vi "energy_list.vi"(10 "list_peak_energies":string[][](array[string]), 11 "List Calibration":T2[](array[typedef]) {"Select Line" items=["Ka1", "Ka2", "Kb1", "La1", "La2", "Lb1", "Lb2", "Lg1"]; "Select Element" items=["Li", "Be", "B", "C", "N", "O", "F", "Ne", "Na", "Mg", "Al", "Si", "P", "S", "Cl", "Ar", "K", "Ca", "Sc", "Ti", "V", "Cr", "Mn", "Fe", "Co", "Ni", "Cu", "Zn", "Ga", "Ge", "As", "Se", "Br", "Kr", "Rb", "Sr", "Y", "Zr", "Nb", "Mo", "Tc", "Ru", "Rh", "Pd", "Ag", "Cd", "In", "Sn", "Sb", "Te", "I", "Xe", "Cs", "Ba", "La", "Ce", "Pr", "Nd", "Pm", "Sm", "Eu", "Gd", "Tb", "Dy", "Ho", "Er", "Tm", "Yb", "Lu", "Hf", "Ta", "W", "Re", "Os", "Ir", "Pt", "Au", "Hg", "Tl", "Pb", "Bi", "Po", "At", "Rn", "Fr", "Ra", "Ac", "Th", "Pa", "U", "Np", "Pu", "Am"]}) -> (1 "Check":bool[](array[boolean]), 2 "to calibrate":T1, 3 "List Calibration Out":T2[](array[typedef]) {"Select Line" items=["Ka1", "Ka2", "Kb1", "La1", "La2", "Lb1", "Lb2", "Lg1"]; "Select Element" items=["Li", "Be", "B", "C", "N", "O", "F", "Ne", "Na", "Mg", "Al", "Si", "P", "S", "Cl", "Ar", "K", "Ca", "Sc", "Ti", "V", "Cr", "Mn", "Fe", "Co", "Ni", "Cu", "Zn", "Ga", "Ge", "As", "Se", "Br", "Kr", "Rb", "Sr", "Y", "Zr", "Nb", "Mo", "Tc", "Ru", "Rh", "Pd", "Ag", "Cd", "In", "Sn", "Sb", "Te", "I", "Xe", "Cs", "Ba", "La", "Ce", "Pr", "Nd", "Pm", "Sm", "Eu", "Gd", "Tb", "Dy", "Ho", "Er", "Tm", "Yb", "Lu", "Hf", "Ta", "W", "Re", "Os", "Ir", "Pt", "Au", "Hg", "Tl", "Pb", "Bi", "Po", "At", "Rn", "Fr", "Ra", "Ac", "Th", "Pa", "U", "Np", "Pu", "Am"]})   [LabVIEW 2023]
uses:
  control/calib.ctl
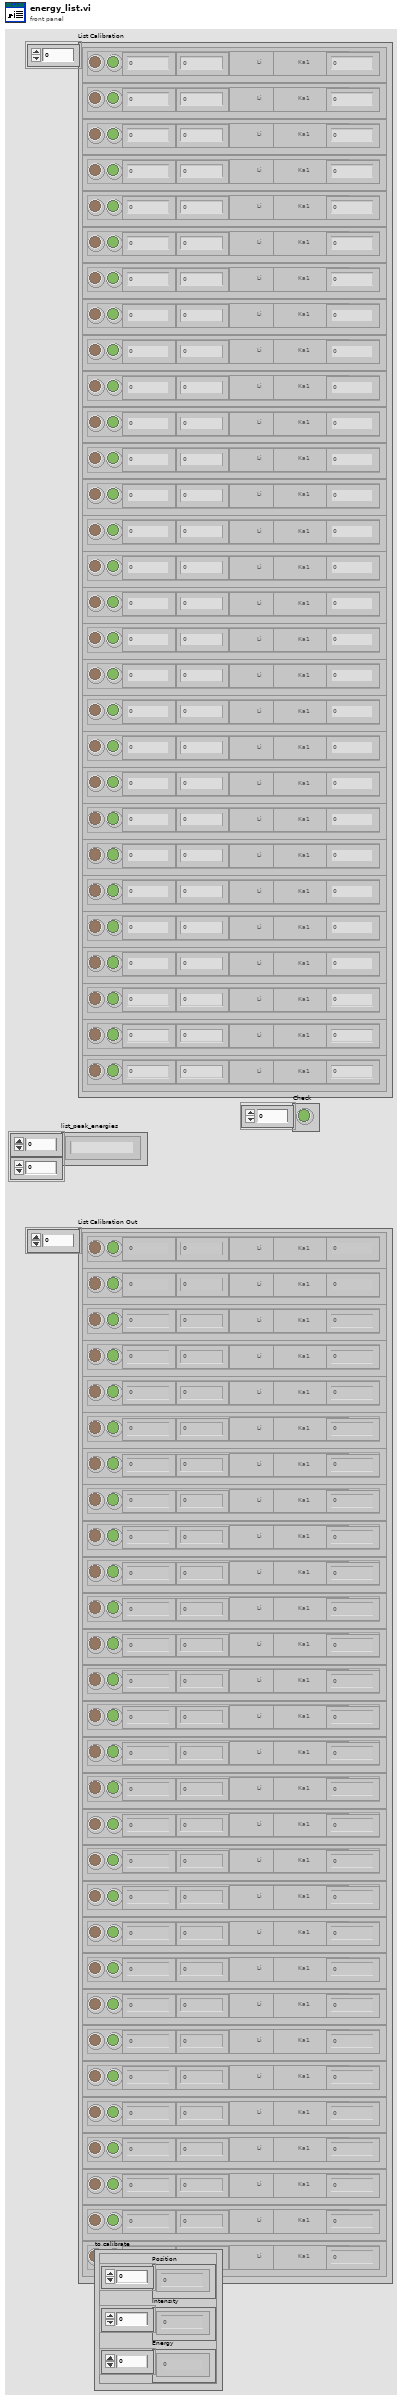
[diagram p1: front panel]
types:
  T1 = cluster{"Position":dbl[], "Intensity":dbl[], "Energy":dbl[]}
  T2 = typedef "calib.ctl" = cluster{"select":bool, "Position":dbl, "Select Element":u16, "Select Line":u16, "Intensity":dbl, "Energy":dbl, "best":bool}
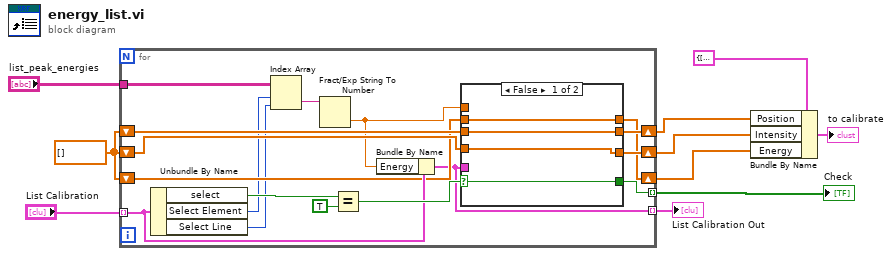
[diagram p0: block diagram]
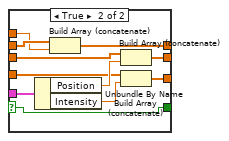
[diagram p2: hidden frame]
diagram:
  w8 = dbl[] []
  n1 = for {
    tunnel: "List Calibration" -> [w24] mode=indexing
    shift-right: [w22] -> w3
    shift-left: w8 -> [w20]
    shift-right: [w23] -> w4
    shift-left: w8 -> [w21]
    shift-right: [w19] -> w2
    shift-left: w8 -> [w18]
    tunnel: [w17] -> w6 mode=indexing
    tunnel: "list_peak_energies" -> [w14]
    tunnel: [w11] -> w7 mode=indexing
    n2 = Unbundle By Name(w24) -> ("select"=w27:bool, "Select Element"=w16:u16, "Select Line"=w15:u16)
    n3 = Index Array(array=w14, index (row)=w16, index (col)=w15) -> (element=w13:string)
    n4 = Fract/Exp String To Number(string=w13) -> (number=w12:dbl)  [unwired: 3 in, 1 out]
    n5 = Equal?(x=w27, y=TRUE) -> (x = y?=w25:bool)
    n6 = Bundle By Name(cluster=w24, "Energy"=w12) -> (w11:T2)
    n7 = case shown="False" w25 {
      selector: w25 -> [w28 w34]
      tunnel: [w31 w40] -> w23
      tunnel: [w30 w39] -> w22
      tunnel: w21 -> [w31 w38]
      tunnel: w20 -> [w30 w37]
      tunnel: [w29 w36] -> w19
      tunnel: w18 -> [w29 w35]
      tunnel: [w28 w34] -> w17
      tunnel: w12 -> [_ w33]
      tunnel: w11 -> [_ w32]
      frame False {
      }
      frame True {
        n8 = Unbundle By Name(w32) -> ("Position"=w41:dbl, "Intensity"=w42:dbl)
        n9 = Build Array (concatenate)(w35, w33) -> (w36:dbl[])
        n10 = Build Array (concatenate)(w38, w41) -> (w40:dbl[])
        n11 = Build Array (concatenate)(w37, w42) -> (w39:dbl[])
      }
    }
  }
  "List Calibration Out" <- w7
  "Check" <- w6
  n12 = Bundle By Name(cluster=T1 {"Position"=[], "Intensity"=[], "Energy"=[]}, "Position"=w4, "Intensity"=w3, "Energy"=w2) -> (→"to calibrate":T1)
